vi "DHE_DRV_read_frame_time.vi"(0 "fd":i32, 11 "error in (no error)":errorcluster) -> (4 "fd out":i32, 8 "return value":i32, 15 "error out":errorcluster)   [LabVIEW 2016]
doc: "This VI closes the I/O interface with the instrument."
uses:
  c/lib/libarcDHE.so
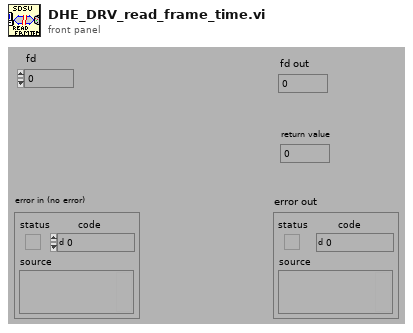
[diagram p1: front panel]
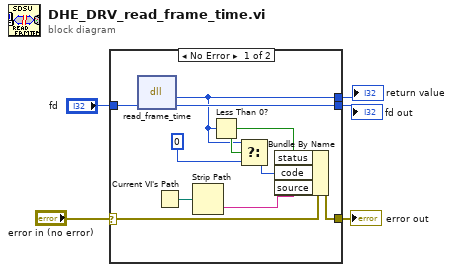
[diagram p0: block diagram]
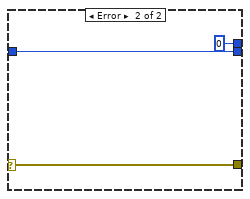
[diagram p2: hidden frame]
diagram:
  n1 = case shown="No Error" "error in (no error)" {
    selector: "error in (no error)" -> [w10 w16]
    tunnel: "fd" -> [w15 w18]
    tunnel: [w7 0] -> w4
    tunnel: [w12 w16] -> w3
    tunnel: [w11 w18] -> w2
    frame No Error {
      n2 = dll-call lib="home/simager/panview/PAN/Modules/SDSU/private/c/lib/libarcDHE.so" fn="read_frame_time"("fd"=w15) -> (w7:i32, "fd"=w11:i32)  [unwired: 3 in, 2 out]
      n3 = Current VI's Path() -> (path=w14:path)
      n4 = Strip Path(path=w14) -> (name=w13:string)  [unwired: 1 out]
      n5 = Less Than 0?(x=w7) -> (x < 0?=w9:bool)
      n6 = Select(t=w7, s=w9, f=0) -> (s? t:f=w8:i32)
      n7 = Bundle By Name(cluster=w10, "status"=w9, "code"=w8, "source"=w13) -> (w12:errorcluster)
    }
    frame Error {
    }
  }
  "error out" <- w3
  "return value" <- w4
  "fd out" <- w2
